vi "Query Variant.vi"(0 "VCluster in":variant, 1 "Reference Variant":variant, 5 "basePath in":string, 7 "pathList":string[](array[string]), 9 "Reorder\nqueried\nvariants?":bool, 11 "error IO":errorcluster, 12 "Include\n2D array?":bool) -> (4 "VCluster\n out":variant, 6 "Error Message":string, 8 "No error?":bool, 15 "error out":errorcluster)   [LabVIEW 2015]
doc: "The input array of strings represent the <b>JSON paths</b> to specific elements in the JSON string. These elements are accessed through the path input and the output is provided in the form of <b>VCluster</b> (the bundled form of the input path elements). \nFurthermore, you may use the <b>Variant to Data</b> SubVI to convert back the Variant to the required Cluster type you want."
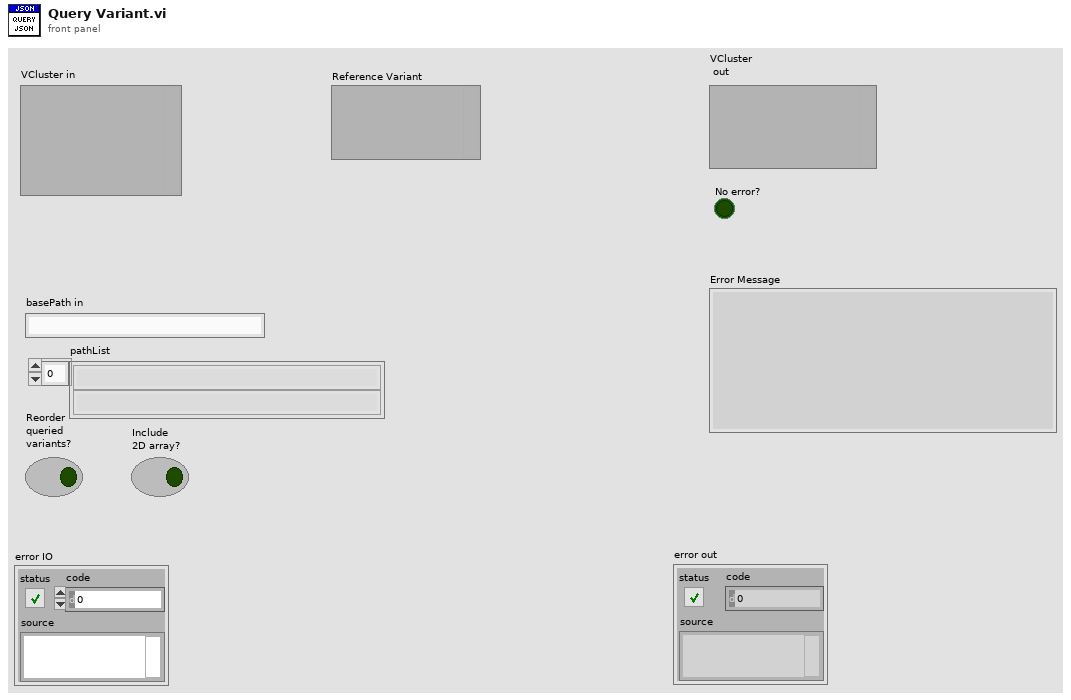
[diagram p1: front panel]
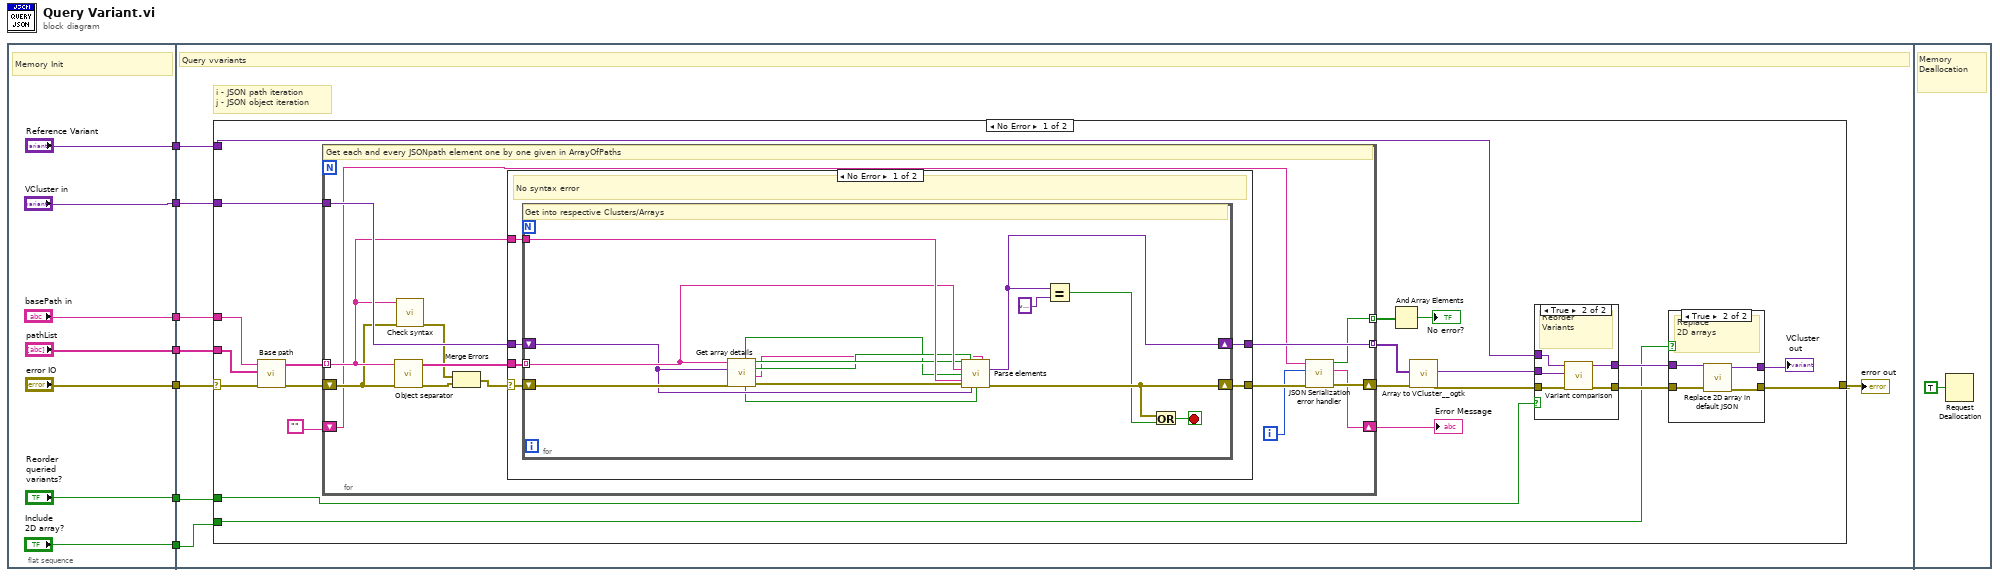
[diagram p0: block diagram]
diagram:
  n1 = flat-sequence {
    tunnel: ["Reference Variant"] -> w7
    tunnel: ["VCluster in"] -> w6
    tunnel: ["basePath in"] -> w5
    tunnel: ["pathList"] -> w4
    tunnel: ["error IO"] -> w3
    tunnel: ["Reorder\nqueried\nvariants?"] -> w2
    tunnel: ["Include\n2D array?"] -> w1
    tunnel: w7 -> [w21]
    tunnel: w6 -> [w20]
    tunnel: w5 -> [w19]
    tunnel: w4 -> [w18]
    tunnel: w3 -> [w17]
    tunnel: w2 -> [w16]
    tunnel: w1 -> [w15]
    frame #0 {
      # "Memory Init"
    }
    frame #1 {
      # "i - JSON path iteration\nj - JSON object iteration"
      # "Query vvariants"
      n2 = case shown="No Error" w17 {
        selector: w17 -> [w37 w93]
        tunnel: [w31 w93] -> w22
        tunnel: w18 -> [w34 _]
        tunnel: w16 -> [w33 _]
        tunnel: w21 -> [w27 _]
        tunnel: w15 -> [w28 _]
        tunnel: w19 -> [w26 _]
        tunnel: w20 -> [w25 _]
        frame No Error {
          n3 = call "Base path.vi"("error in (no error)"=w37, "pathList"=w34, "basePath in"=w26) -> ("error out"=w41:errorcluster, "pathArray out"=w40:string[])  [unwired: 7 in]
          n4 = for {
            tunnel: w40 -> [w67] mode=indexing
            shift-right: [w65] -> w43
            shift-left: w41 -> [w63]
            tunnel: [w69] -> w42 mode=indexing
            shift-right: [w64] -> w39
            shift-left: "" -> [w57]
            tunnel: w25 -> [w68]
            tunnel: [w58] -> w24 mode=indexing
            i -> [w59]
            # "Get each and every JSONpath element one by one given in ArrayOfPaths"
            n5 = call "Object separator.vi"("error in (no error)"=w63, "json path in"=w67) -> ("error out"=w61:errorcluster, "output array of keys"=w70:string[])  [unwired: 8 in]
            n6 = call "Check syntax.vi"("error in"=w63, "<single path ele>"=w67) -> ("error out"=w62:errorcluster)  [unwired: 9 in]
            n7 = Merge Errors(w62, w61) -> (w60:errorcluster)
            n8 = case shown="No Error" w60 {
              selector: w60 -> [w71 w92]
              tunnel: w70 -> [w76 _]
              tunnel: [w75 _] -> w69
              tunnel: w68 -> [w74 _]
              tunnel: w67 -> [w73 _]
              tunnel: [w72 w92] -> w66
              frame No Error {
                # "No syntax error"
                n9 = for {
                  tunnel: w76 -> [w88] mode=indexing
                  shift-right: [w90] -> w75
                  shift-left: w74 -> [w79]
                  shift-right: [w87] -> w72
                  shift-left: w71 -> [w89]
                  tunnel: w73 -> [w91]
                  stop <- w85 stop-if-true
                  # "Get into respective Clusters/Arrays"
                  n10 = call "Get array details.vi"("error in (no error)"=w89, "Current obejct"=w79, "Separate object string"=w88) -> ("error out"=w83:errorcluster, "Required object"=w80:string, "Non-index array?"=w81:bool, "Is array?"=w82:bool, "Array contained cluster?"=w77:bool, "Complete Array?"=w78:bool)  [unwired: 3 in]
                  n11 = call "Parse elements.vi"("Is array?"=w82, "Non indexed arrays?"=w81, "Required object"=w80, "Single path element"=w88, "Complete Array?"=w78, "JSON Path"=w91, "error in (no error)"=w83, "Variant"=w79, "Array contained cluster?"=w77) -> ("VArray"=w90:variant, "error out"=w87:errorcluster)  [unwired: 5 in]
                  n12 = Equal?(x=w90, y=variant) -> (x = y?=w86:bool)
                  n13 = Or(x=w87, y=w86) -> (x .or. y?=w85:bool)
                }
              }
              frame Error {
                # "Syntax error"
              }
            }
            n14 = call "JSON Serialization error handler.vi"("error in (no error)"=w66, "Error check path index"=w59, "Previous path error string"=w57) -> ("error out"=w65:errorcluster, "Concaternated error\nstring"=w64:string, "No error?"=w58:bool)  [unwired: 5 in, 1 out]
          }
          "Error Message" <- w39
          n15 = And Array Elements(Boolean array=w24) -> (logical AND=→"No error?":bool)
          n16 = call <userlib>:"Array to VCluster__ogtk.vi"("error in (no error)"=w43, "Array"=w42) -> ("error out"=w36:errorcluster, "VCluster"=w35:variant)  [unwired: 8 in]
          n17 = case shown="True" w33 {
            tunnel: w36 -> [w51 w56]
            tunnel: [w51 w54] -> w32
            tunnel: w35 -> [w50 w53]
            tunnel: [w50 w55] -> w30
            tunnel: w27 -> [_ w52]
            frame False {
            }
            frame True {
              # "Reorder\nVariants"
              n18 = call "Variant comparison.vi"("error in (no error)"=w56, "Data Variant"=w53, "Reference Variant"=w52) -> ("error out"=w54:errorcluster, "Output VData"=w55:variant)  [unwired: 7 in]
            }
          }
          n19 = case shown="True" w28 {
            tunnel: w32 -> [w44 w49]
            tunnel: [w44 w48] -> w31
            tunnel: w30 -> [w45 w46]
            tunnel: [w45 w47] -> w29
            frame False {
            }
            frame True {
              # "Replace\n2D arrays"
              n20 = call "Replace 2D array in default JSON.vi"("error in (no error)"=w49, "VCluster with Array of Arrays"=w46) -> ("error out"=w48:errorcluster, "VCluster with replaced 2D Array"=w47:variant)  [unwired: 8 in]
            }
          }
          "VCluster\n out" <- w29
        }
        frame Error {
        }
      }
      "error out" <- w22
    }
    frame #2 {
      # "Memory Deallocation"
      n21 = Request Deallocation(TRUE ("flag")) -> ()
    }
  }
